vi "GEOM_VAR_DETECTORS_uncorr_unbin.vi"(9 "Action":T2, 10 "det in":cluster{"name":string, "detectors":T1[]}[](array[cluster])) -> (2 "det out":cluster{"name":string, "detectors":T1[]}[](array[cluster]))   [LabVIEW 2016]
uses:
  GEOM_VAR_action.ctl
  GEOM_DetSummaryStruct.ctl
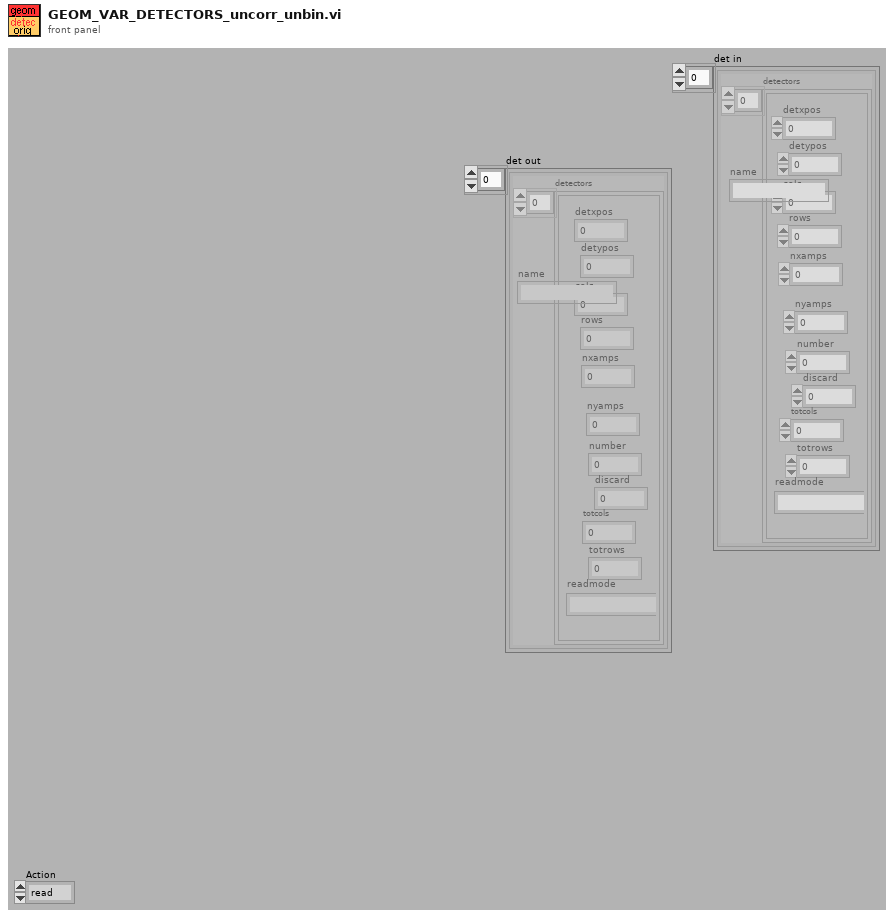
[diagram p1: front panel]
types:
  T1 = typedef "GEOM_DetSummaryStruct.ctl" = cluster{"detxpos":i32, "detypos":i32, "cols":i32, "rows":i32, "nxamps":i32, "nyamps":i32, "number":i32, "discard":i32, "totcols":i32, "totrows":i32, "readmode":string}
  T2 = typedef "GEOM_VAR_action.ctl" = enum16{"read", "write"}
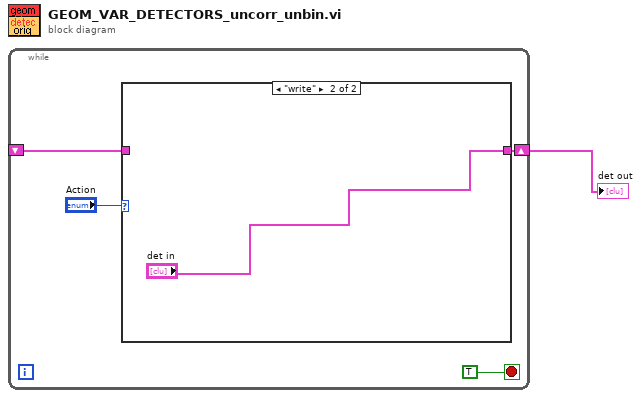
[diagram p0: block diagram]
diagram:
  n1 = while {
    shift-right: [w4] -> w1
    shift-left: _ -> [w3]
    stop <- TRUE stop-if-true
    n2 = case shown="\"write\"" "Action" {
      tunnel: [w6 "det in"] -> w4
      tunnel: w3 -> [w6 _]
      frame "read", Default {
      }
      frame "write" {
      }
    }
  }
  "det out" <- w1
